vi "Battery Charge.vi"() -> ()   [LabVIEW 2019]
panel:
  out "Under-voltage Warning (<3,5V)":bool
  out "Over-voltage Warning (>4,2V)":bool
  out "Low Capacity Warning (<20%)":bool
  in  "Stop Button":bool
  out "XY Graph":cluster{dbl[], dbl[]}(graph)
  out "output variable":dbl
  in  "Input Voltage":dbl(slide) scale=3.27..4.2
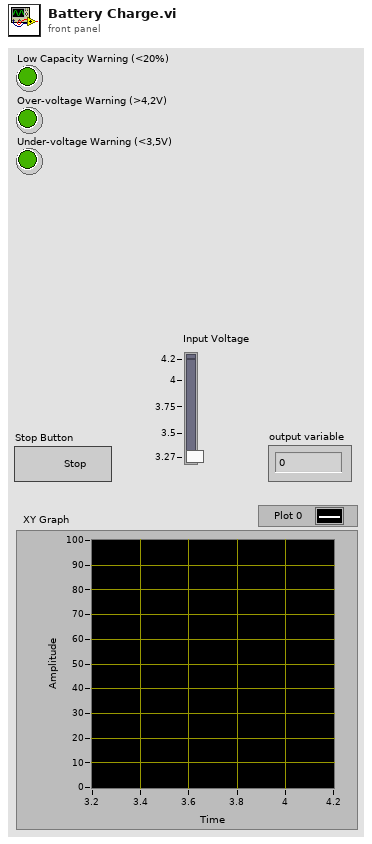
[diagram p1: front panel]
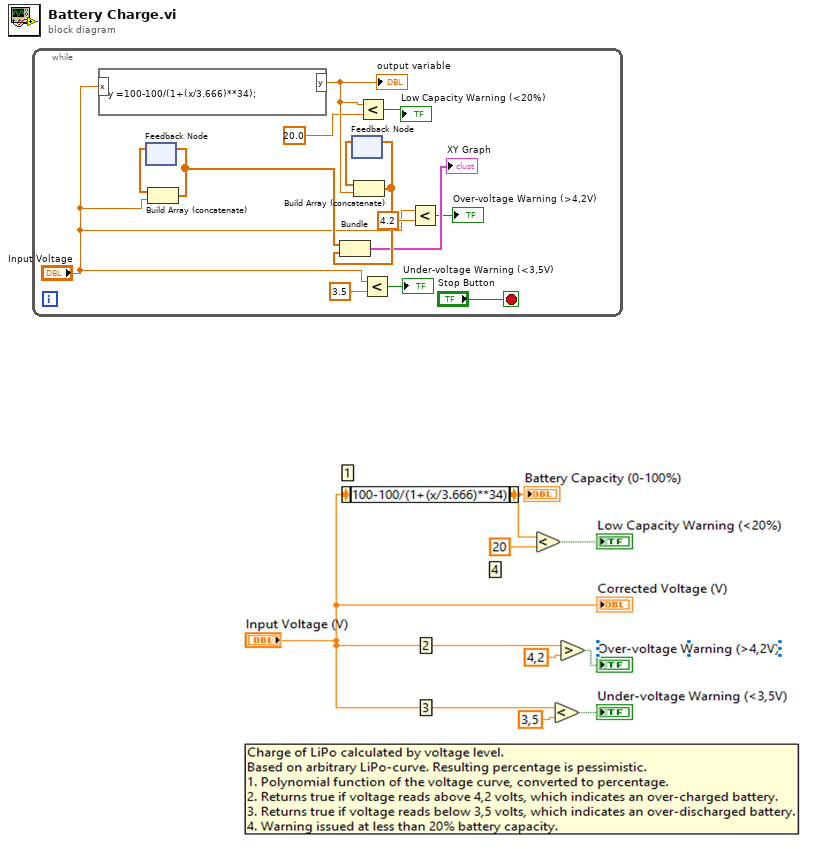
[diagram p0: block diagram]
diagram:
  n1 = while {
    stop <- "Stop Button" stop-if-true
    n2 = formula code="y =100-100/(1+(x/3.666)**34);"("x"="Input Voltage") -> ("y"=w8:dbl)
    "output variable" <- w8
    n3 = feedback #1() -> (w14:dbl[])  [unwired: 1 in]
    n4 = Build Array (concatenate)(w14, "Input Voltage") -> (w12:dbl[])
    n5 = feedback-in #1(w12) -> ()
    n6 = feedback #2() -> (w13:dbl[])  [unwired: 1 in]
    n7 = Build Array (concatenate)(w13, w8) -> (w11:dbl[])
    n8 = Bundle(w12, w11) -> (→"XY Graph":cluster{dbl[], dbl[]})  [unwired: 1 in]
    n9 = feedback-in #2(w11) -> ()
    n10 = Less?(x=w8, y=20.0) -> (x < y?=→"Low Capacity Warning (<20%)":bool)
    n11 = Less?(x="Input Voltage", y=3.5) -> (x < y?=→"Under-voltage Warning (<3,5V)":bool)
    n12 = Less?(x="Input Voltage", y=4.2) -> (x < y?=→"Over-voltage Warning (>4,2V)":bool)
  }
